vi "Condicionales.vi"() -> ()   [LabVIEW 2018]
panel:
  in  "stop":bool
  out "Contar min":i32
  out "Contar May":i32
  out "Boolean 3":bool
  out "Boolean 2":bool
  out "Contraseñas":u8[](array[numeric])
  out "coerced(x)":i32
  out "Boolean":bool
  in  "contraseña":string
  in  "usuario":string
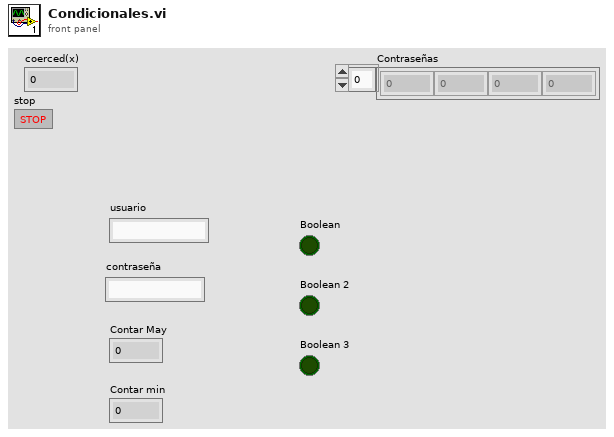
[diagram p1: front panel]
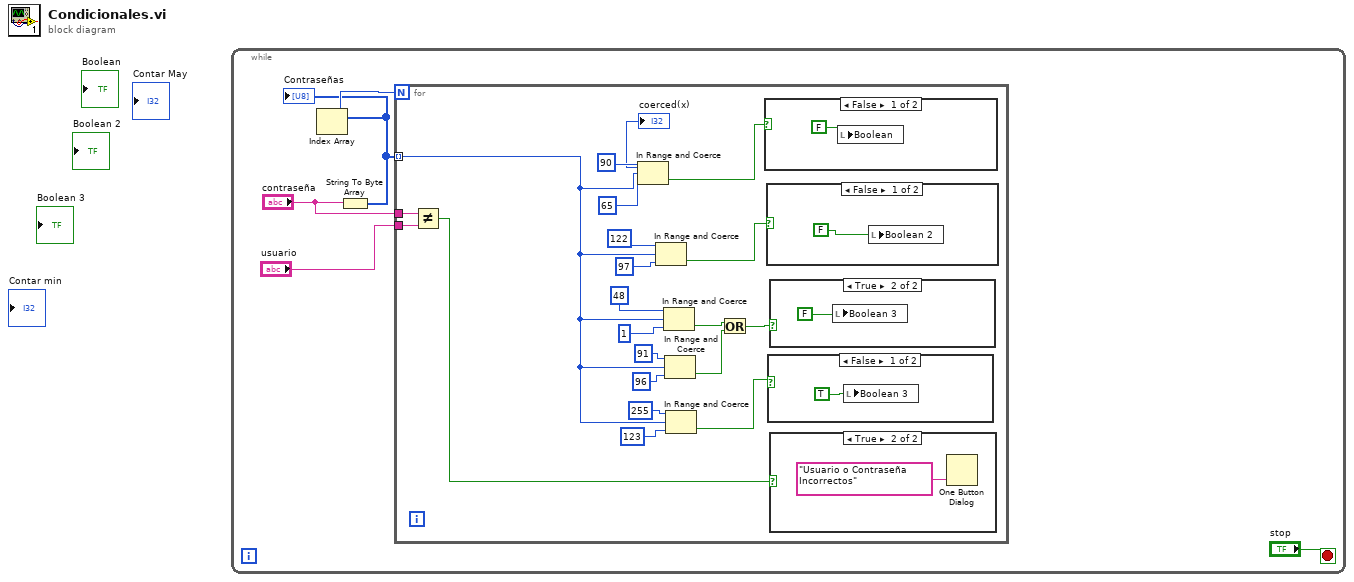
[diagram p0: block diagram]
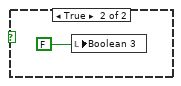
[diagram p3: hidden frame]
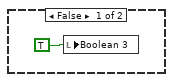
[diagram p4: hidden frame]
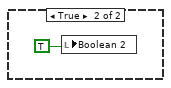
[diagram p5: hidden frame]
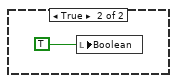
[diagram p6: hidden frame]
diagram:
  n1 = while {
    stop <- "stop" stop-if-true
    n2 = String To Byte Array(string="contraseña") -> (unsigned byte array=w4:u8[])
    "Contraseñas" <- w4
    n3 = Index Array(array=w4) -> (element=w5:u8)  [unwired: 1 in]
    n4 = for {
      N: w5 -> [_]
      tunnel: w4 -> [w7] mode=indexing
      tunnel: "usuario" -> [w11]
      tunnel: "contraseña" -> [w10]
      n5 = Not Equal?(x=w10, y=w11) -> (x != y?=w9:bool)
      n6 = In Range and Coerce(upper limit=90, x=w7, lower limit=65) -> (coerced(x)=→"coerced(x)":i32, In Range?=w14:bool)
      n7 = In Range and Coerce(upper limit=122, x=w7, lower limit=97) -> (In Range?=w15:bool)  [unwired: 1 out]
      n8 = In Range and Coerce(upper limit=48, x=w7, lower limit=1) -> (In Range?=w13:bool)  [unwired: 1 out]
      n9 = In Range and Coerce(upper limit=u8 91, x=w7, lower limit=u8 96) -> (In Range?=w12:bool)  [unwired: 1 out]
      n10 = In Range and Coerce(upper limit=u8 255, x=w7, lower limit=u8 123) -> (In Range?=w6:bool)  [unwired: 1 out]
      n11 = Or(x=w13, y=w12) -> (x .or. y?=w8:bool)
      n12 = case shown="False" w14 {
        frame False {
          n13 = local write "Boolean"(FALSE) -> ()
        }
        frame True {
          n14 = local write "Boolean"(TRUE) -> ()
        }
      }
      n15 = case shown="False" w15 {
        frame False {
          n16 = local write "Boolean 2"(FALSE) -> ()
        }
        frame True {
          n17 = local write "Boolean 2"(TRUE) -> ()
        }
      }
      n18 = case shown="False" w6 {
        frame False {
          n19 = local write "Boolean 3"(TRUE) -> ()
        }
        frame True {
          n20 = local write "Boolean 3"(FALSE) -> ()
        }
      }
      n21 = case shown="True" w8 {
        frame False {
          n22 = local write "Boolean 3"(TRUE) -> ()
        }
        frame True {
          n23 = local write "Boolean 3"(FALSE) -> ()
        }
      }
      n24 = case shown="True" w9 {
        frame False {
        }
        frame True {
          n25 = One Button Dialog(message="Usuario o Contraseña      Incorrectos") -> ()  [unwired: 1 in, 1 out]
        }
      }
    }
  }
